vi "FirstOrderSystem.vi"(7 "T":dbl, 9 "T_s":dbl, 10 "u_k-1":dbl, 11 "y_k-1":dbl) -> (3 "y_k":dbl)   [LabVIEW 2020]
doc: "First order discrete system.\n\nT is the time constant.\nT_s is the sampling time."
uses:
  <vilib>/express/express arith-compare/Formula/XNode/ExpressFormulaBlockNode.xnode
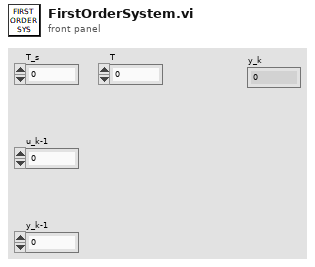
[diagram p1: front panel]
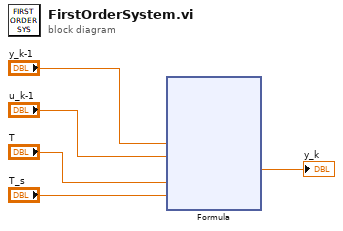
[diagram p0: block diagram]
diagram:
  n1 = xnode "Formula"("y"="y_k-1", "u"="u_k-1", "T"="T", "Ts"="T_s") -> ("Result"=→"y_k":dbl)  [unwired: 1 in, 1 out]
